vi "Create Message Getter (from Template).vi"(7 "replace string in template":string="package_templatemessage", 8 "error in (no error)":errorcluster, 9 "template VI name":string="Get package_templatemessage.vi", 10 "RPC Message Name":string, 11 "RPC Messages Folder (ProjectItem) in":refnum<vi>) -> (0 "error out":errorcluster, 1 "Created?":bool, 2 "Getter VI out":refnum<vi>, 3 "RPC Messages Folder (ProjectItem) out":refnum<vi>)   [LabVIEW 2019, in "gRPC Template Creation Utility.lvlib"]
uses:
  gRPC Template Creation Utility.lvlib
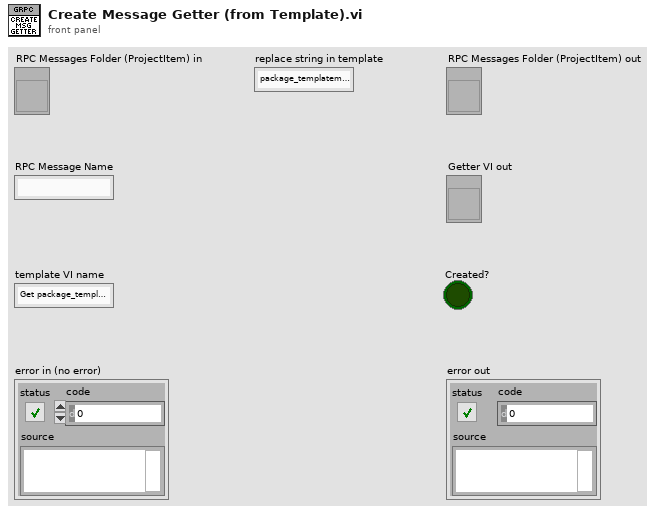
[diagram p1: front panel]
types:
  T1 = enum32{"invalid VI type", "Standard VI", "Control VI", "Global VI", "Polymorphic VI", "Configuration VI", "SubSystem", "Facade VI", "Method VI"}
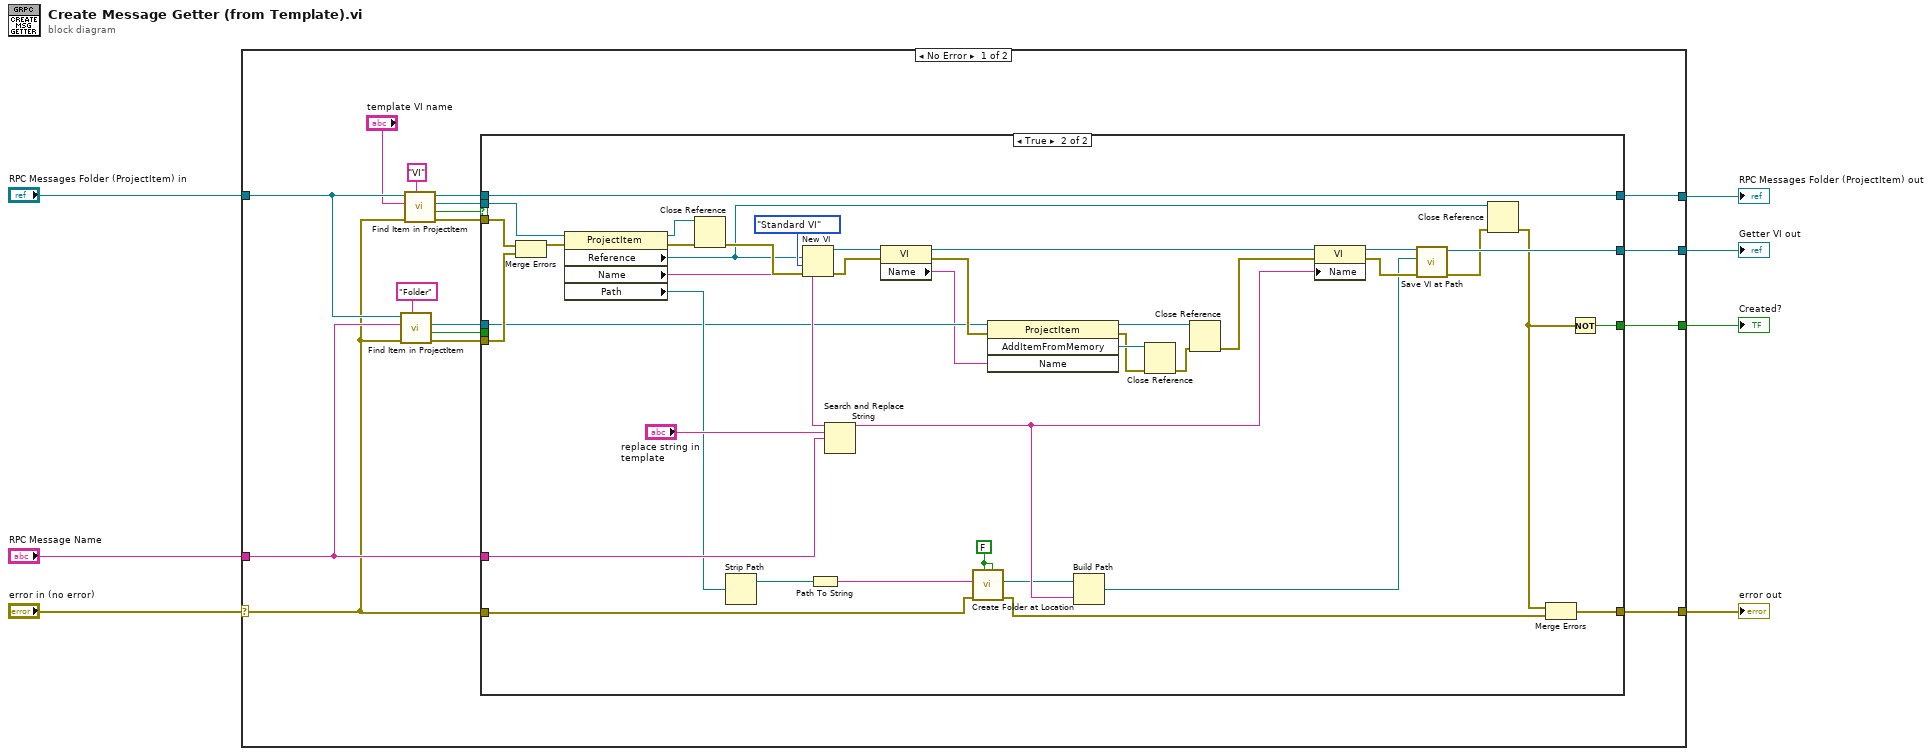
[diagram p0: block diagram]
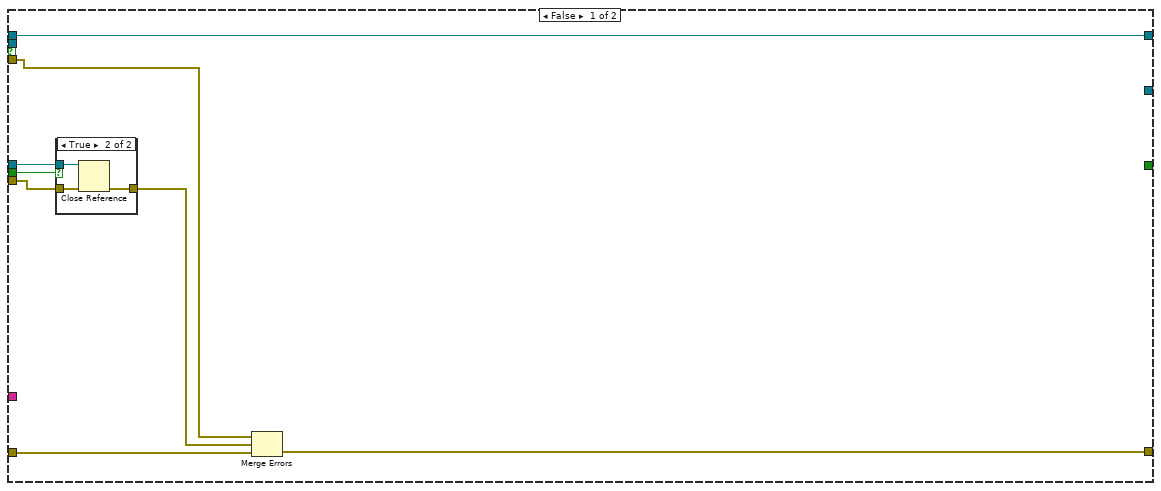
[diagram p2: hidden frame]
diagram:
  n1 = case shown="No Error" "error in (no error)" {
    selector: "error in (no error)" -> [w13 w77]
    tunnel: "RPC Message Name" -> [w24 _]
    tunnel: "RPC Messages Folder (ProjectItem) in" -> [w23 w78]
    tunnel: [w22 w77] -> w5
    tunnel: [w10 w78] -> w4
    tunnel: [w19 _] -> w3
    tunnel: [w9 _] -> w1
    frame No Error {
      n2 = call "Find Item in ProjectItem.vi"("Item Type"="Folder", "error in (no error)"=w13, "Name"=w24, "ProjectItem in"=w23) -> ("error out"=w21:errorcluster, "Found ?"=w8:bool, "Item Refnum out"=w18:refnum<vi>)  [unwired: 4 in, 1 out]
      n3 = call "Find Item in ProjectItem.vi"("Item Type"="VI", "error in (no error)"=w13, "Name"="template VI name", "ProjectItem in"=w23) -> ("error out"=w20:errorcluster, "Found ?"=w12:bool, "Item Refnum out"=w17:refnum<vi>, "ProjectItem out"=w11:refnum<vi>)  [unwired: 4 in]
      n4 = case shown="True" w12 {
        tunnel: w24 -> [_ w76]
        tunnel: [w27 w72] -> w22
        tunnel: w21 -> [w31 w70]
        tunnel: w20 -> [w25 w68]
        tunnel: [_ w66] -> w19
        tunnel: w18 -> [w30 w54]
        tunnel: w17 -> [_ w49]
        tunnel: w13 -> [w28 w48]
        tunnel: w11 -> [w32 w47]
        tunnel: [w32 w47] -> w10
        tunnel: [_ w44] -> w9
        tunnel: w8 -> [w26 _]
        frame False {
          n5 = case shown="True" w26 {
            tunnel: w31 -> [w33 w36]
            tunnel: w30 -> [_ w35]
            tunnel: [w33 w34] -> w29
            frame False {
            }
            frame True {
              n6 = Close Reference(reference=w35, error in (no error)=w36) -> (error out=w34:errorcluster)
            }
          }
          n7 = Merge Errors(w25, w29, w28) -> (w27:errorcluster)
        }
        frame True {
          w67 = FALSE ("Use Relative (F)")
          n8 = Merge Errors(w68, w70) -> (w69:errorcluster)
          n9 = property class="ProjectItem"(reference=w49, error in=w69) -> (reference out=w75:refnum<vi>, error out=w73:errorcluster, "Reference"=w38:refnum<vi>, "Name"=w58:string, "Path"=w56:path)
          n10 = Close Reference(reference=w75, error in (no error)=w73) -> (error out=w74:errorcluster)
          n11 = Strip Path(path=w56) -> (stripped path=w37:path)  [unwired: 1 out]
          n12 = New VI(8:w74, 9:T1."Standard VI" ("vi type (standard vi)"), 10:w38) -> (0:w52:errorcluster, 3:w50:refnum<vi>)  [unwired: 1 in, 3 out]
          n13 = Path To String(path=w37) -> (string=w55:string)
          n14 = Search and Replace String(input string=w58, search string="replace string in template", replace string=w76) -> (result string=w62:string)  [unwired: 5 in, 3 out]
          n15 = property class="VI"(reference=w50, error in=w52) -> (reference out=w59:refnum<vi>, error out=w60:errorcluster, "Name"=w53:string)
          n16 = call "Create Folder at Location.vi"("Override existing (F)"=w67, "Use Relative (F)"=w67, "Error In"=w48, "Path"=w55) -> ("Error Out"=w71:errorcluster, "Full path out"=w61:path)  [unwired: 5 in, 1 out]
          n17 = invoke class="ProjectItem" method="AddItemFromMemory"(reference=w54, error in=w60, "Name"=w53) -> (reference out=w46:refnum<vi>, error out=w42:errorcluster, "AddItemFromMemory"=w43:refnum<vi>)  [unwired: 1 in, 1 out]
          n18 = Build Path(base path=w61, name or relative path=w62) -> (appended path=w64:path)
          n19 = Close Reference(reference=w43, error in (no error)=w42) -> (error out=w41:errorcluster)
          n20 = Close Reference(reference=w46, error in (no error)=w41) -> (error out=w45:errorcluster)
          n21 = property class="VI"(reference=w59, error in=w45, "Name"=w62) -> (reference out=w63:refnum<vi>, error out=w65:errorcluster)
          n22 = call "Save VI at Path.vi"("error in (no error)"=w65, "Path"=w64, "VI in"=w63) -> ("error out"=w40:errorcluster, "VI out"=w66:refnum<vi>)  [unwired: 6 in, 1 out]
          n23 = Close Reference(reference=w38, error in (no error)=w40) -> (error out=w39:errorcluster)
          n24 = Merge Errors(w39, w71) -> (w72:errorcluster)
          n25 = Not(x=w39) -> (.not. x?=w44:bool)
        }
      }
    }
    frame Error {
    }
  }
  "error out" <- w5
  "RPC Messages Folder (ProjectItem) out" <- w4
  "Getter VI out" <- w3
  "Created?" <- w1
